vi "Goto Wave (close slits).vi"(8 "error in (no error)":errorcluster, 10 "Target Wavelength":dbl[unit], 11 "Spectrometer Triax 550 in":refnum<class "Spectrometer Triax 550.lvclass">) -> (0 "error out":errorcluster, 2 "Actual Wavelength":dbl[unit], 3 "Spectrometer Triax 550 out":refnum<class "Spectrometer Triax 550.lvclass">)   [LabVIEW 2017, in "Spectrometer Triax 550.lvclass"]
doc: "Close the slits before moving the wavelength, then restore the slits. This could prevent crossing a spectral line which might overload the photomultiplier tube."
uses:
  Spectrometer Triax 550.lvclass
  JY-SPEX-TRIAX/controls.llb/Slits.ctl
  JY-SPEX-TRIAX/JY-SPEX-TRIAX.lvlib
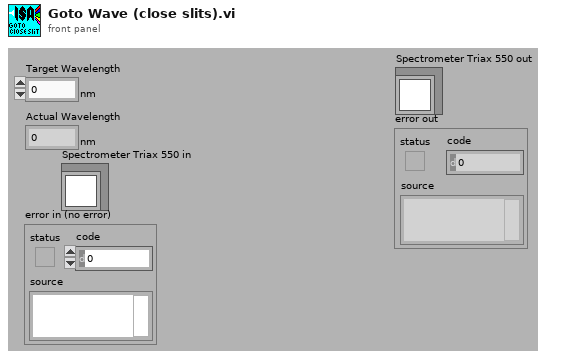
[diagram p1: front panel]
types:
  T1 = typedef "JY-SPEX-TRIAX.lvlib/Slits.ctl" = enum16{"0 (Front/Axial Entrance)", "1 (Side/Lateral Entrance)", "2 (Front/Axial Exit)", "3 (Side/Lateral Exit)"}
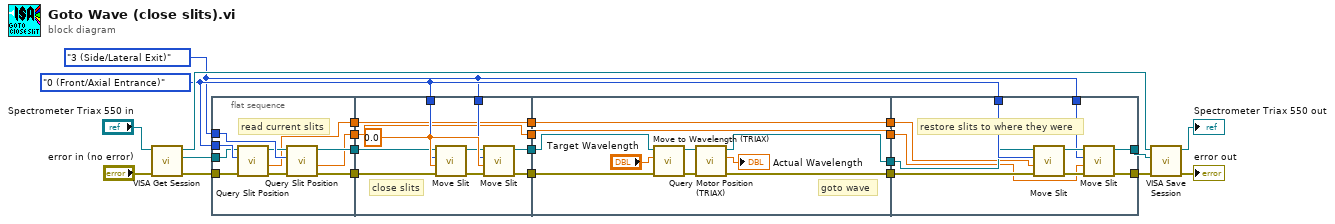
[diagram p0: block diagram]
diagram:
  w15 = Slits."0 (Front/Axial Entrance)" ("Slit (Front/Axial Entrance)")
  w14 = Slits."3 (Side/Lateral Exit)" ("Slit (Front/Axial Entrance)")
  n1 = call-dynamic "VISA Get Session.vi"("error in (no error)"="error in (no error)", "Instrument.lvclass in"="Spectrometer Triax 550 in") -> ("error out"=w11:errorcluster, "VISA Resource Name"=w16:refnum<visa-resource-name>, "Instrument.lvclass out"=w22:refnum<class "Spectrometer Triax 550.lvclass">)  [unwired: 7 out]
  n2 = flat-sequence {
    tunnel: w14 -> [w33]
    tunnel: w15 -> [w32]
    tunnel: [w31] -> w18
    tunnel: [w28] -> w17
    tunnel: w16 -> [w27]
    tunnel: w11 -> [w26]
    tunnel: [w25] -> w4
    tunnel: [w24] -> w3
    tunnel: w14 -> [w41]
    tunnel: w15 -> [w40]
    tunnel: w18 -> [w39]
    tunnel: w17 -> [w38]
    tunnel: [w37] -> w10
    tunnel: [w36] -> w7
    tunnel: [w35] -> w5
    tunnel: w4 -> [w35]
    tunnel: w3 -> [w34]
    tunnel: [w34] -> w2
    tunnel: w10 -> [w52]
    tunnel: [w51] -> w9
    tunnel: [w50] -> w8
    tunnel: w7 -> [w49]
    tunnel: [w46] -> w6
    tunnel: w5 -> [w46]
    tunnel: w2 -> [w45]
    tunnel: [w45] -> w1
    tunnel: w15 -> [w63]
    tunnel: w14 -> [w62]
    tunnel: [w60] -> w13
    tunnel: [w59] -> w12
    tunnel: w9 -> [w58]
    tunnel: w8 -> [w57]
    tunnel: w6 -> [w56]
    tunnel: w1 -> [w55]
    frame #0 {
      # "read current slits"
      n3 = call "Query Slit Position.vi"("error in (no error)"=w26, "Slit (Front/Axial Entrance)"=w32, "VISA resource name"=w27) -> ("error out"=w30:errorcluster, "Slit Position"=w24:dbl[unit], "VISA resource name out"=w29:refnum<visa-resource-name>)  [unwired: 1 in, 5 out]
      n4 = call "Query Slit Position.vi"("error in (no error)"=w30, "Slit (Front/Axial Entrance)"=w33, "VISA resource name"=w29) -> ("error out"=w31:errorcluster, "Slit Position"=w25:dbl[unit], "VISA resource name out"=w28:refnum<visa-resource-name>)  [unwired: 1 in, 5 out]
    }
    frame #1 {
      w43 = dbl[unit] 0.0 ("Desired Slit Position")
      # "close slits"
      n5 = call "Move Slit.vi"("error in (no error)"=w39, "Desired Slit Position"=w43, "Slit (Front/Axial Entrance)"=w40, "VISA resource name"=w38) -> ("error out"=w44:errorcluster, "VISA resource name out"=w42:refnum<visa-resource-name>)  [unwired: 1 in, 5 out]
      n6 = call "Move Slit.vi"("error in (no error)"=w44, "Desired Slit Position"=w43, "Slit (Front/Axial Entrance)"=w41, "VISA resource name"=w42) -> ("error out"=w36:errorcluster, "VISA resource name out"=w37:refnum<visa-resource-name>)  [unwired: 1 in, 5 out]
    }
    frame #2 {
      # "goto wave"
      n7 = call "Move to Wavelength (TRIAX).vi"("error in (no error)"=w49, "Target wavelength"="Target Wavelength", "VISA resource name"=w52) -> ("error out"=w54:errorcluster, "VISA resource name out"=w53:refnum<visa-resource-name>)  [unwired: 1 in, 6 out]
      n8 = call "Query Motor Position (TRIAX).vi"("error in (no error)"=w54, "VISA resource name"=w53) -> ("error out"=w50:errorcluster, "wavelength"=→"Actual Wavelength":dbl[unit], "VISA resource name out"=w51:refnum<visa-resource-name>)  [unwired: 1 in, 6 out]
    }
    frame #3 {
      # "restore slits to where they were"
      n9 = call "Move Slit.vi"("error in (no error)"=w57, "Desired Slit Position"=w55, "Slit (Front/Axial Entrance)"=w63, "VISA resource name"=w58) -> ("error out"=w61:errorcluster, "VISA resource name out"=w64:refnum<visa-resource-name>)  [unwired: 1 in, 5 out]
      n10 = call "Move Slit.vi"("error in (no error)"=w61, "Desired Slit Position"=w56, "Slit (Front/Axial Entrance)"=w62, "VISA resource name"=w64) -> ("error out"=w59:errorcluster, "VISA resource name out"=w60:refnum<visa-resource-name>)  [unwired: 1 in, 5 out]
    }
  }
  n11 = call-dynamic "VISA Save Session.vi"("error in (no error)"=w12, "VISA Resource Name"=w13, "Instrument.lvclass in"=w22) -> ("error out"=→"error out":errorcluster, "Instrument.lvclass out"=→"Spectrometer Triax 550 out":refnum<class "Spectrometer Triax 550.lvclass">)  [unwired: 7 out]
